vi "Set Instrument Name.vi"(8 "Error In":errorcluster, 10 "Instrument Name":string, 11 "reference in":refnum<class "Instrument Base.lvclass">) -> (0 "Error Out":errorcluster, 3 "reference out":refnum<class "Instrument Base.lvclass">)   [LabVIEW 2023, in "HAL GOOP4.lvlib" / "Instrument Base.lvclass"]
uses:
  Instrument Base.lvclass
  Instrument Base.lvclass/Instrument Base.ctl
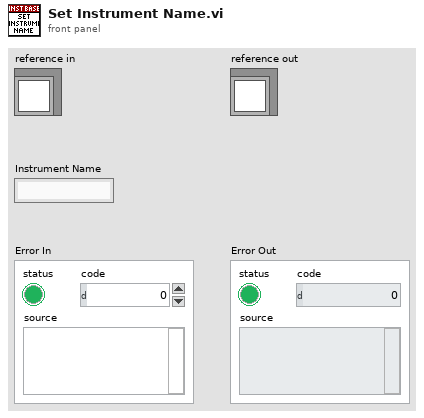
[diagram p1: front panel]
types:
  T1 = typedef "HAL GOOP4.lvlib/Instrument Base.lvclass/ObjectAttributes.ctl" = cluster{"Instr Identifier":string, "IConfigure":refnum<class "IConfigure.lvclass">}
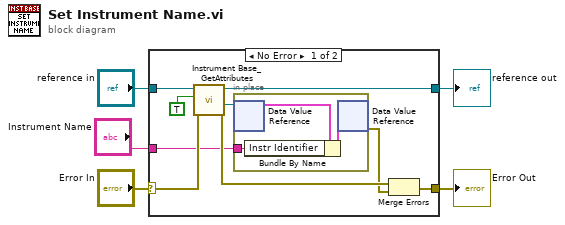
[diagram p0: block diagram]
diagram:
  n1 = case shown="No Error" "Error In" {
    selector: "Error In" -> [w13 w19]
    tunnel: [w14 w19] -> w4
    tunnel: [w10 w18] -> w2
    tunnel: "reference in" -> [w11 w18]
    tunnel: "Instrument Name" -> [w7 _]
    frame No Error {
      n2 = call "Instrument Base_GetAttributes.vi"("Error In"=w13, "OnlyGetDvrReference(False)"=TRUE, "reference in"=w11) -> ("Error Out"=w12:errorcluster, "DataRef"=w8:refnum<data-value>, "reference out"=w10:refnum<class "Instrument Base.lvclass">)  [unwired: 5 in, 1 out]
      n3 = in-place {
        in-place-border: w7 -> [w17]
        n4 = in-place-dvr #1(w8) -> (w16:T1)  [unwired: 1 out]
        n5 = Bundle By Name(cluster=w16, "Instr Identifier"=w17) -> (w15:T1)
        n6 = in-place-dvr #1(w15) -> (w6:errorcluster)  [unwired: 1 out]
      }
      n7 = Merge Errors(w12, w6) -> (w14:errorcluster)
    }
    frame Error {
    }
  }
  "Error Out" <- w4
  "reference out" <- w2
